vi "Bus Interface.vi"(0 "AddressSpace":refnum<class "AddressSpace.lvclass">, 1 "abort":bool, 5 "instruction":T2, 9 "input valid":bool) -> (6 "response":T1, 10 "done":bool, 14 "ready for input":bool)   [LabVIEW 2015, in "QuadEnc.lvlib" / "AddressSpace.lvclass"]
uses:
  AddressSpace.lvclass
  <instrlib>/_niInstr/Instruction Framework/v1/FPGA/Interfaces/Address Space/Address Space Instruction.ctl
  <instrlib>/_niInstr/Instruction Framework/v1/FPGA/Typedefs/Response.ctl
  AddressSpace.lvclass/AddressSpace.ctl
  <vilib>/Utility/error.llb/Clear Errors.vi
  <vilib>/rvi/Emulation/niFpgaSctlEmulationGetInTimedLoop.vi
  <vilib>/rvi/DataTransferAndStorage/Container/Common/niFpgaContainerExecOnDevCompGetState.vi
  <vilib>/rvi/Emulation/niFpgaEmulationIsFPGAContextNoSignature.vi
  <vilib>/rvi/DataTransferAndStorage/Container/Common/niFpgaContainerGetUniqueNameForEmu.vi
  <vilib>/rvi/Memory/Memory_Emulation/niFpgaMemoryEmulationCacheClearOnFirstRun.vi
  <vilib>/rvi/Memory/Memory_Emulation/nirvimemoryEmulationManagerCache_MakeExclusive.vi
  <vilib>/rvi/Memory/Memory_Emulation/niFpgaMemoryEmulationValidateCache.vi
  <vilib>/rvi/Memory/Memory_Emulation/nirvimemoryEmulationManagerCache_InsertValue.vi
  <vilib>/rvi/Memory/Memory_Emulation/nirvimemoryEmulationManagerCache_ReleaseExclusive.vi
  <vilib>/rvi/Memory/Memory_Emulation/nirvimemoryEmulationManagerCache_GetValue.vi
  <vilib>/rvi/Memory/Memory_Emulation/nirvimemoryEmulationManagerCache_SetValue.vi
  <vilib>/rvi/Emulation/niFpgaProcessEmulError.vi
  <vilib>/rvi/DataTransferAndStorage/Container/XNode/niFpgaContainer.xnode
  <vilib>/rvi/DataTransferAndStorage/Register/Emulation/niFpgaRegisterEmulationRefIn.vi
  <instrlib>/_niInstr/Instruction Framework/v1/FPGA/Typedefs/niInstr Instruction Framework v1 FPGA.lvlib
  QuadEnc.lvlib
  <instrlib>/_niInstr/Instruction Framework/v1/FPGA/Interfaces/Address Space/Address Space.lvclass
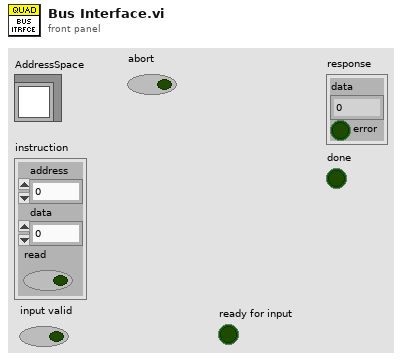
[diagram p1: front panel]
types:
  T1 = typedef "niInstr Instruction Framework v1 FPGA.lvlib/Response.ctl" = cluster{"data":u64, "error":bool}
  T2 = typedef "niInstr Instruction Framework Interfaces v1 FPGA.lvlib/Address Space.lvclass/Address Space Instruction.ctl" = cluster{"address":u32, "data":u64, "read":bool}
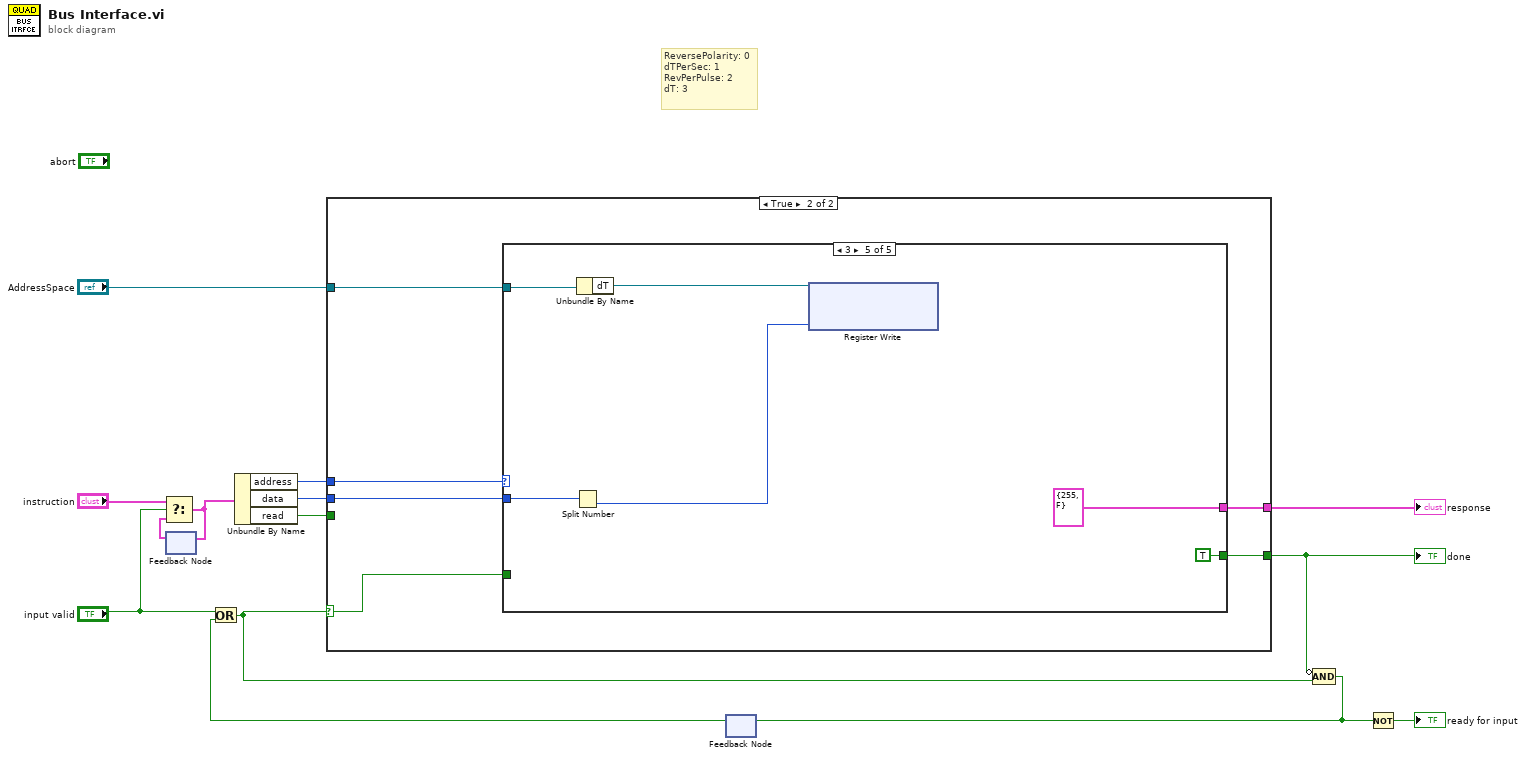
[diagram p0: block diagram]
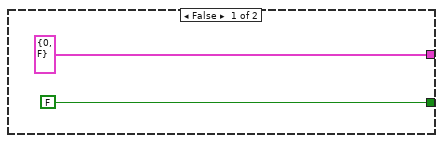
[diagram p2: hidden frame]
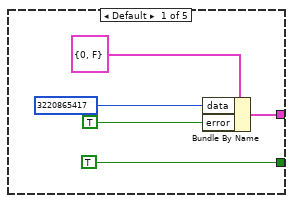
[diagram p3: hidden frame]
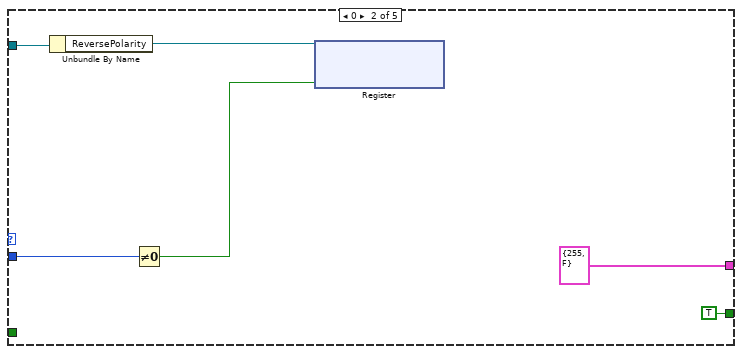
[diagram p4: hidden frame]
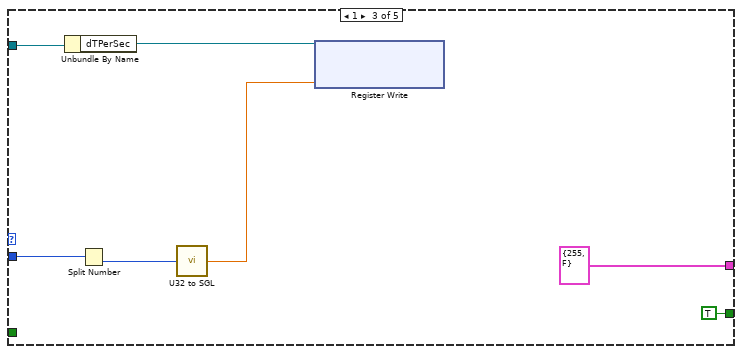
[diagram p5: hidden frame]
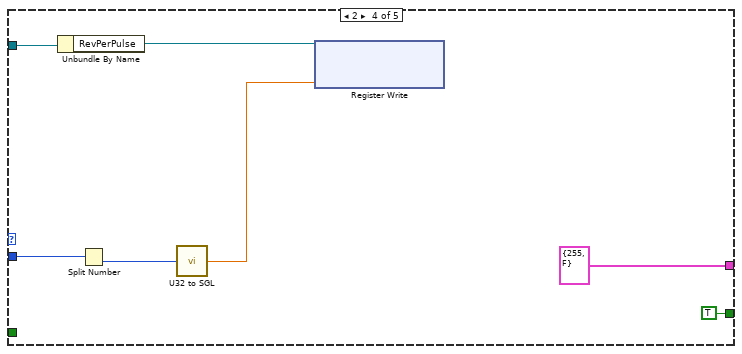
[diagram p6: hidden frame]
diagram:
  # "ReversePolarity: 0\ndTPerSec: 1\nRevPerPulse: 2\ndT: 3"
  n1 = feedback #1() -> (w14:T2)  [unwired: 1 in]
  n2 = Select(t="instruction", s="input valid", f=w14) -> (s? t:f=w13:T2)
  n3 = feedback-in #1(w13) -> ()
  n4 = Unbundle By Name(w13) -> ("address"=w10:u32, "data"=w11:u64, "read"=w12:bool)
  n5 = feedback #2() -> (w7:bool)  [unwired: 1 in]
  n6 = Or(x="input valid", y=w7) -> (x .or. y?=w8:bool)
  n7 = case shown="True" w8 {
    selector: w8 -> [_ w17]
    tunnel: w12 -> [_ _]
    tunnel: w10 -> [_ w22]
    tunnel: w11 -> [_ w21]
    tunnel: [T1 {"data"=0, "error"=FALSE} ("response") w20] -> w3
    tunnel: [FALSE ("Output Valid") w19] -> w2
    tunnel: "AddressSpace" -> [_ w18]
    frame False {
    }
    frame True {
      n8 = case shown="3" w22 {
        tunnel: w21 -> [_ w29 w36 w43 w49]
        tunnel: [w24 T1 {"data"=255, "error"=FALSE} ("response") T1 {"data"=255, "error"=FALSE} ("response") T1 {"data"=255, "error"=FALSE} ("response") T1 {"data"=255, "error"=FALSE} ("response")] -> w20
        tunnel: [TRUE ("done") TRUE ("done") TRUE ("done") TRUE ("done") TRUE ("done")] -> w19
        tunnel: w18 -> [_ w33 w40 w47 w53]
        tunnel: w17 -> [_ _ _ _ _]
        frame Default {
          n9 = Bundle By Name(cluster=T1 {"data"=0, "error"=FALSE} ("response"), "data"=u64 3220865417, "error"=TRUE) -> (w24:T1)
        }
        frame 0 {
          n10 = Unbundle By Name(w33) -> ("ReversePolarity"=w30:refnum<k21>)
          n11 = Not Equal To 0?(x=w29) -> (x != 0?=w28:bool)
          n12 = xnode "Register"("Data"=w28, "Register In"=w30) -> ()  [unwired: 1 out]
        }
        frame 1 {
          n13 = Unbundle By Name(w40) -> ("dTPerSec"=w37:refnum<k21>)
          n14 = Split Number(x=w36) -> (lo(x)=w35:u32)  [unwired: 1 out]
          n15 = call "U32 to SGL.vi"("U32"=w35) -> ("SGL"=w34:sgl)  [unwired: 4 in]
          n16 = xnode "Register Write"("Data"=w34, "Register In"=w37) -> ()  [unwired: 1 out]
        }
        frame 2 {
          n17 = Unbundle By Name(w47) -> ("RevPerPulse"=w44:refnum<k21>)
          n18 = Split Number(x=w43) -> (lo(x)=w42:u32)  [unwired: 1 out]
          n19 = call "U32 to SGL.vi"("U32"=w42) -> ("SGL"=w41:sgl)  [unwired: 4 in]
          n20 = xnode "Register Write"("Data"=w41, "Register In"=w44) -> ()  [unwired: 1 out]
        }
        frame 3 {
          n21 = Split Number(x=w49) -> (lo(x)=w48:u32)  [unwired: 1 out]
          n22 = Unbundle By Name(w53) -> ("dT"=w50:refnum<k21>)
          n23 = xnode "Register Write"("Data"=w48, "Register In"=w50) -> ()  [unwired: 1 out]
        }
      }
    }
  }
  "done" <- w2
  "response" <- w3
  n24 = Compound Arithmetic op=AND(invert w2, w8) -> (w9:bool)
  n25 = feedback-in #2(w9) -> ()
  n26 = Not(x=w9) -> (.not. x?=→"ready for input":bool)
